vi "AB_GetNextLabel.vi"(7 "label type (buildSpec)":T2, 8 "error in (no error)":errorcluster, 9 "default name":string="My Application", 10 "supplied name":string="My Application", 11 "buildObject":T1) -> (0 "error out":errorcluster, 3 "New label":string)   [LabVIEW 2020]
uses:
  <vilib>/AppBuilder/AB_LabelType.ctl
  <resource>/Framework/Providers/API/ItemRef.ctl
  <vilib>/AppBuilder/RW_Project/AB_RW_Project_PropBag_Action.ctl
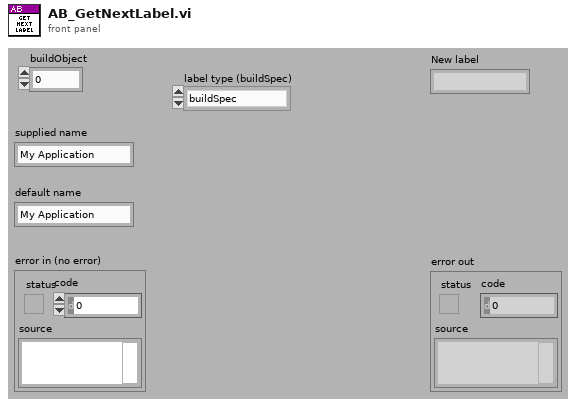
[diagram p1: front panel]
types:
  T1 = typedef "ItemRef.ctl" = u64
  T2 = typedef "AB_LabelType.ctl" = enum16{"buildSpec", "targetFilename"}
  T3 = typedef "AB_RW_Project_PropBag_Action.ctl" = enum16{"read", "write", "clear", "readPrevious", "writePrevious", "clearPrevious"}
  T4 = typedef "AB_RW_Project_TargetFile_Data.ctl" = cluster{"targetfileName":string, "targetfileGUID":string, "enableDebugging":bool, "productName":string, "legalCopyright":string, "companyName":string, "internalName":string, "fileDescription":string, "eng_topLevelVI_DestinationPaths":path[], "fastFileFormat":bool, "versionIndependent":bool}
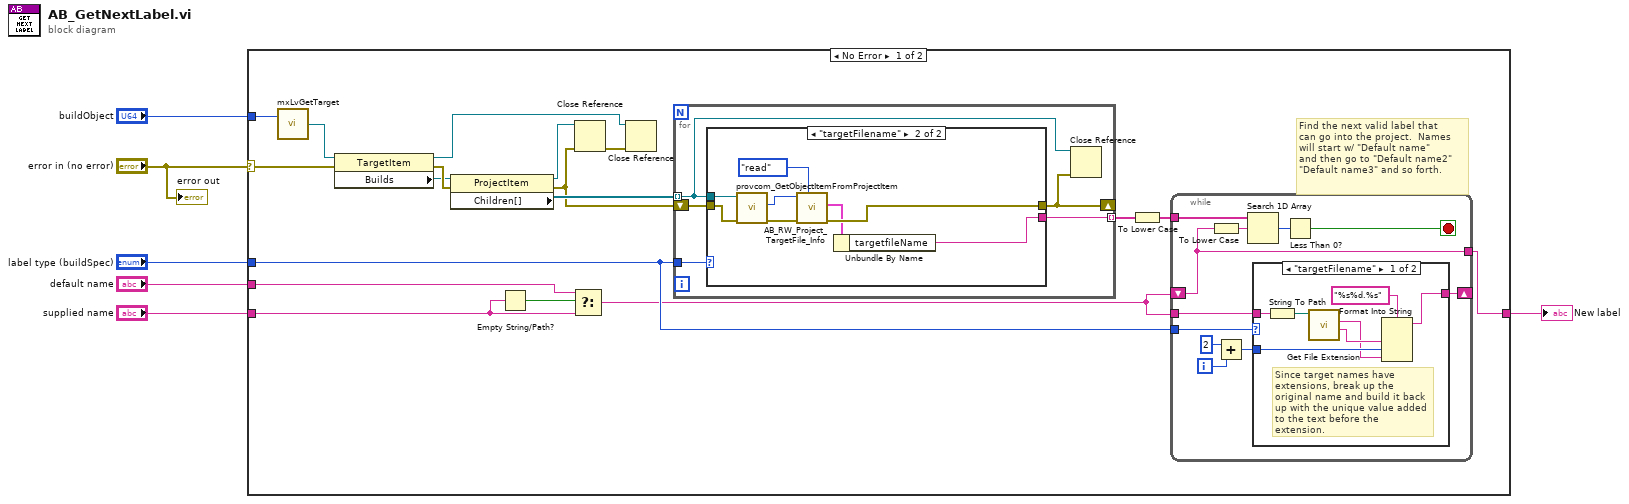
[diagram p0: block diagram]
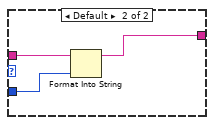
[diagram p2: hidden frame]
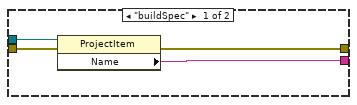
[diagram p3: hidden frame]
diagram:
  n1 = case shown="No Error" "error in (no error)" {
    selector: "error in (no error)" -> [w24 _]
    tunnel: "supplied name" -> [w22 _]
    tunnel: [w23 _] -> w5
    tunnel: "label type (buildSpec)" -> [w21 _]
    tunnel: "buildObject" -> [w20 _]
    tunnel: "default name" -> [w19 _]
    frame No Error {
      # "Find the next valid label that\ncan go into the project.  Names\nwill start w/ \"Default name\"\nand then go to \"Default name2\"\n\"Default name3\" and so forth."
      n2 = call <resource>:"mxLvGetTarget.vi"("Item"=w20) -> ("Target"=w10:refnum<vi>)  [unwired: 1 in, 2 out]
      n3 = property class="TargetItem"(reference=w10, error in=w24) -> (reference out=w9:refnum<vi>, error out=w17:errorcluster, "Builds"=w15:refnum<vi>)
      n4 = property class="ProjectItem"(reference=w15, error in=w17) -> (reference out=w13:refnum<vi>, error out=w14:errorcluster, "Children[]"=w18:refnum<vi>[])
      n5 = Empty String/Path?(string/path=w22) -> (empty?=w8:bool)
      n6 = Select(t=w19, s=w8, f=w22) -> (s? t:f=w7:string)
      n7 = Close Reference(reference=w13, error in (no error)=w14) -> (error out=w11:errorcluster)
      n8 = Close Reference(reference=w9, error in (no error)=w11) -> ()  [unwired: 1 out]
      n9 = for {
        tunnel: w18 -> [w46] mode=indexing
        shift-right: [w47] -> _
        shift-left: w14 -> [w50]
        tunnel: [w49] -> w16 mode=indexing
        tunnel: w21 -> [w48]
        n10 = case shown="\"targetFilename\"" w48 {
          tunnel: w46 -> [w54 w62]
          tunnel: w50 -> [w53 w61]
          tunnel: [w52 w57] -> w47
          tunnel: [w51 w55] -> w49
          frame "buildSpec" {
            n11 = property class="ProjectItem"(reference=w54, error in=w53) -> (error out=w52:errorcluster, "Name"=w51:string)  [unwired: 1 out]
          }
          frame "targetFilename" {
            n12 = call <resource>:"provcom_GetObjectItemFromProjectItem.vi"("error in (no error)"=w61, "ProjectItem"=w62) -> ("error out"=w60:errorcluster, "ObjectItem"=w59:T1)  [unwired: 7 in, 1 out]
            n13 = call <vilib>:"AB_RW_Project_TargetFile_Info.vi"("action"=AB_RW_Project_PropBag_Action."read", "error in (no error)"=w60, "Object In"=w59) -> ("error out"=w57:errorcluster, "targetfile info"=w56:T4)  [unwired: 6 in, 1 out]
            n14 = Unbundle By Name(w56) -> ("targetfileName"=w55:string)
          }
        }
        n15 = Close Reference(reference=w46, error in (no error)=w47) -> ()  [unwired: 1 out]
      }
      n16 = To Lower Case(string=w16) -> (all lower case string=w12:string[])
      n17 = while {
        tunnel: w12 -> [w33]
        shift-right: [w28] -> _
        shift-left: w7 -> [w30]
        tunnel: [w30] -> w23
        tunnel: w7 -> [w26]
        tunnel: w21 -> [w25]
        i -> [w32]
        stop <- w27 stop-if-true
        n18 = To Lower Case(string=w30) -> (all lower case string=w34:string)
        n19 = Add(x=2, y=w32) -> (x+y=w29:i32)
        n20 = Search 1D Array(1D array=w33, element=w34) -> (index of element=w35:i32)  [unwired: 1 in]
        n21 = case shown="\"targetFilename\"" w25 {
          tunnel: w29 -> [w37 w45]
          tunnel: [w39 w44] -> w28
          tunnel: w26 -> [w41 w43]
          frame "targetFilename" {
            # "Since target names have extensions, break up the original name and build it back up with the unique value added to the text before the extension."
            n22 = String To Path(string=w41) -> (path=w42:path)
            n23 = call <vilib>:"Get File Extension.vi"("file"=w42) -> ("filename without extension"=w38:string, "lowercase file extension"=w36:string)  [unwired: 6 in, 3 out]
            n24 = Format Into String(format string="%s%d.%s", w38, w37, w36) -> (resulting string=w39:string)  [unwired: 2 in, 1 out]
          }
          frame Default {
            n25 = Format Into String(initial string=w43, w45) -> (resulting string=w44:string)  [unwired: 2 in, 1 out]
          }
        }
        n26 = Less Than 0?(x=w35) -> (x < 0?=w27:bool)
      }
    }
    frame Error {
    }
  }
  "New label" <- w5
  "error out" <- "error in (no error)"
